vi "modbus通信示例程序-bili.vi"() -> ()   [LabVIEW 2020]
uses:
  <vilib>/Instr/_visa.llb/VISA Configure Serial Port (Instr).vi
panel:
  in  "baud rate":u32=9600 caption="波特率"
  in  "写入数值":i16
  out "读取缓冲区 2":string
  out "读取到的值":i16
  out "读取缓冲区":string
  in  "VISA resource name":refnum<visa-resource-name> caption="选择串口"
  in  "写入参数":bool
  in  "读取参数":bool
  # "modbus通信示例程序"
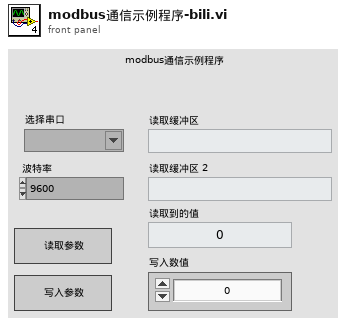
[diagram p1: front panel]
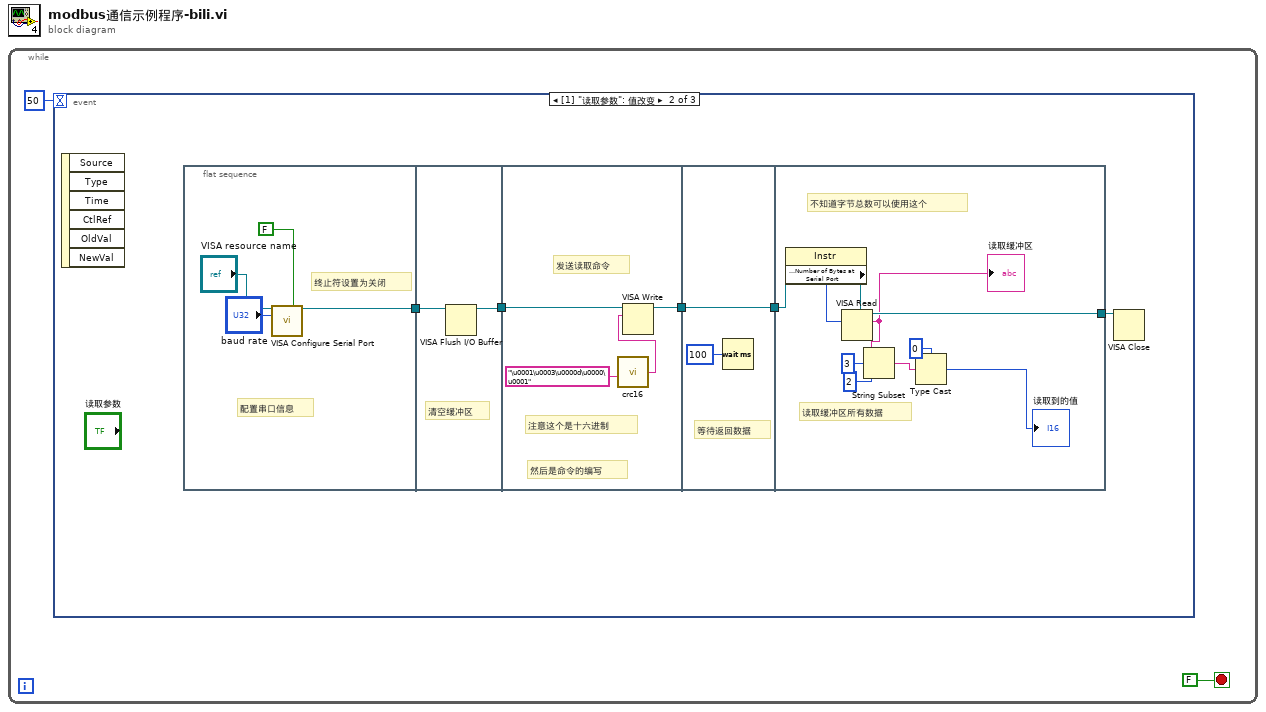
[diagram p0: block diagram]
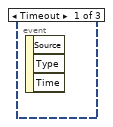
[diagram p2: hidden frame]
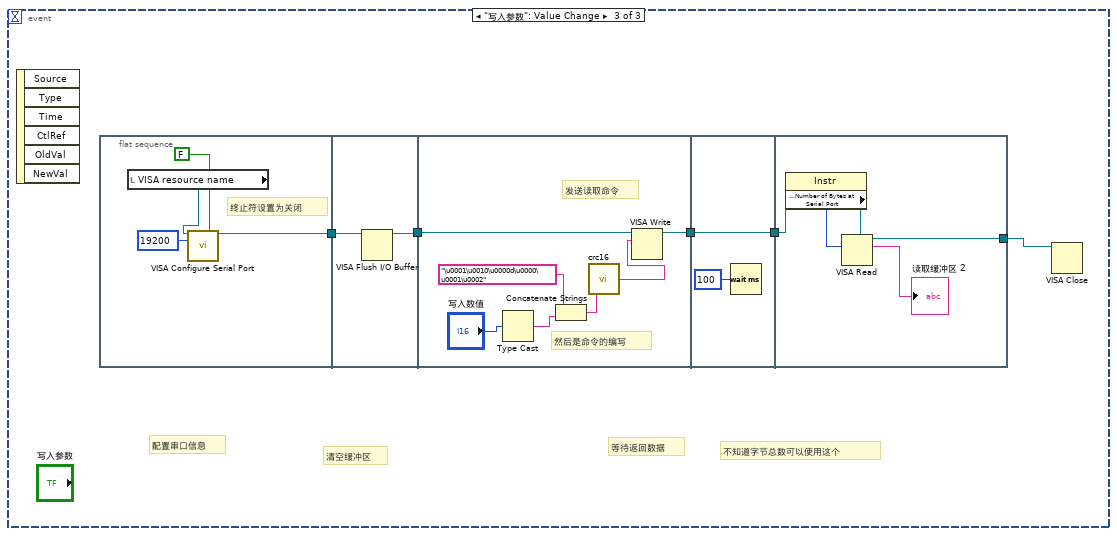
[diagram p3: hidden frame]
diagram:
  n1 = while {
    stop <- FALSE stop-if-true
    n2 = event shown="[1] \"读取参数\": 值改变" {
      selector: _ -> [_ _ _]
      dyn-events: _ -> [_ _ _]
      timeout: 50 -> [_ _ _]
      event Timeout {
        n3 = event-data() -> ()  [unwired: 1 in, 3 out]
      }
      event "读取参数": Value Change {
        n4 = event-data() -> ()  [unwired: 1 in, 6 out]
        n5 = flat-sequence {
          tunnel: [w11] -> w7
          tunnel: w7 -> [w13]
          tunnel: [w12] -> w6
          tunnel: w6 -> [w17]
          tunnel: [w16] -> w5
          tunnel: w5 -> [w19]
          tunnel: [w19] -> w4
          tunnel: w4 -> [w28]
          tunnel: [w29] -> w3
          frame #0 {
            # "配置串口信息"
            # "终止符设置为关闭"
            n6 = call-poly "VISA Configure Serial Port"("VISA resource name"="VISA resource name", "Enable Termination\nChar (T)"=FALSE ("Enable Termination\nChar (T)"), "baud rate (9600)"="baud rate") -> ("VISA resource name out"=w11:refnum<visa-resource-name>)  [unwired: 11 in, 1 out]
          }
          frame #1 {
            # "清空缓冲区"
            n7 = VISA Flush I/O Buffer(VISA resource name=w13) -> (VISA resource name out=w12:refnum<visa-resource-name>)  [unwired: 2 in, 1 out]
          }
          frame #2 {
            # "注意这个是十六进制"
            # "然后是命令的编写"
            # "发送读取命令"
            n8 = call "crc16.vi"("寄存器地址"="\u0001\u0003\u0000d\u0000\u0001") -> ("String & CRC-16"=w14:string)
            n9 = VISA Write(VISA resource name=w17, write buffer=w14) -> (VISA resource name out=w16:refnum<visa-resource-name>)  [unwired: 1 in, 2 out]
          }
          frame #3 {
            # "等待返回数据"
            n10 = Wait (ms)(milliseconds to wait=u32 100 ("等待时间（毫秒）")) -> ()  [unwired: 1 out]
          }
          frame #4 {
            # "不知道字节总数可以使用这个"
            # "读取缓冲区所有数据"
            n11 = property class="Instr"(reference=w28) -> (reference out=w27:refnum<visa-resource-name>, "Serial Settings:Number of Bytes at Serial Port"=w26:u32)  [unwired: 1 in, 1 out]
            n12 = VISA Read(VISA resource name=w27, byte count=w26) -> (VISA resource name out=w29:refnum<visa-resource-name>, read buffer=w25:string)  [unwired: 1 in, 2 out]
            "读取缓冲区" <- w25
            n13 = String Subset(string=w25, offset (0)=3 ("偏移量(0)"), length (rest)=2 ("长度（剩余）")) -> (substring=w22:string)
            n14 = Type Cast(type=i16 0, x=w22) -> (*(type *) &x=→"读取到的值":i16)
          }
        }
        n15 = VISA Close(VISA resource name=w3) -> ()  [unwired: 1 in, 1 out]
      }
      event "写入参数": Value Change {
        # "不知道字节总数可以使用这个"
        # "等待返回数据"
        # "清空缓冲区"
        # "配置串口信息"
        n16 = event-data() -> ()  [unwired: 1 in, 6 out]
        n17 = flat-sequence {
          tunnel: [w38] -> w34
          tunnel: w34 -> [w40]
          tunnel: [w39] -> w33
          tunnel: w33 -> [w47]
          tunnel: [w46] -> w32
          tunnel: w32 -> [w49]
          tunnel: [w49] -> w31
          tunnel: w31 -> [w53]
          tunnel: [w54] -> w30
          frame #0 {
            # "终止符设置为关闭"
            n18 = local read "VISA resource name"() -> (w35:refnum<visa-resource-name>)
            n19 = call-poly "VISA Configure Serial Port"("VISA resource name"=w35, "Enable Termination\nChar (T)"=FALSE ("Enable Termination\nChar (T)"), "baud rate (9600)"=u32 19200) -> ("VISA resource name out"=w38:refnum<visa-resource-name>)  [unwired: 11 in, 1 out]
          }
          frame #1 {
            n20 = VISA Flush I/O Buffer(VISA resource name=w40) -> (VISA resource name out=w39:refnum<visa-resource-name>)  [unwired: 2 in, 1 out]
          }
          frame #2 {
            # "然后是命令的编写"
            # "发送读取命令"
            n21 = Type Cast(x="写入数值") -> (*(type *) &x=w42:string)  [unwired: 1 in]
            n22 = Concatenate Strings("\u0001\u0010\u0000d\u0000\u0001\u0002", w42) -> (w41:string)
            n23 = call "crc16.vi"("寄存器地址"=w41) -> ("String & CRC-16"=w45:string)
            n24 = VISA Write(VISA resource name=w47, write buffer=w45) -> (VISA resource name out=w46:refnum<visa-resource-name>)  [unwired: 1 in, 2 out]
          }
          frame #3 {
            n25 = Wait (ms)(milliseconds to wait=u32 100 ("等待时间（毫秒）")) -> ()  [unwired: 1 out]
          }
          frame #4 {
            n26 = property class="Instr"(reference=w53) -> (reference out=w52:refnum<visa-resource-name>, "Serial Settings:Number of Bytes at Serial Port"=w51:u32)  [unwired: 1 in, 1 out]
            n27 = VISA Read(VISA resource name=w52, byte count=w51) -> (VISA resource name out=w54:refnum<visa-resource-name>, read buffer=→"读取缓冲区 2":string)  [unwired: 1 in, 2 out]
          }
        }
        n28 = VISA Close(VISA resource name=w30) -> ()  [unwired: 1 in, 1 out]
      }
    }
  }
